vi "Dac_Output_cam_trig_multiple_clocks.vi"(0 "File to read":path=path "C:/Users/Hannah/Downloads/newcalibration_voice coil input_25msflyback_3075datapoints.txt", 1 "Image acquisition time (ms)":dbl=1000.0, 2 "Delay between frames":dbl=25.0, 3 "Number of lasers":dbl=3.0, 4 "stop":bool, 5 "error in":errorcluster) -> (19 "error out":errorcluster)   [LabVIEW 2020]
uses:
  <vilib>/DAQmx/write.llb/DAQmx Write (Analog Wfm 1Chan NSamp).vi
  <vilib>/Utility/file.llb/Read Delimited Spreadsheet (DBL).vi
  <vilib>/DAQmx/create/channels.llb/DAQmx Create Channel (AO-Voltage-Basic).vi
  <vilib>/DAQmx/configure/timing.llb/DAQmx Timing (Sample Clock).vi
  <vilib>/DAQmx/miscellaneous.llb/DAQmx Fill In Error Info.vi
  <vilib>/DAQmx/create/channels.llb/DAQmx Create Channel (CO-Pulse Generation-Frequency).vi
  <vilib>/DAQmx/configure/timing.llb/DAQmx Timing (Implicit).vi
  <vilib>/DAQmx/create/channels.llb/DAQmx Create Channel (CO-Pulse Generation-Time).vi
  <resource>/objmgr/daqmx.rc
panel:
  out "error out 2":errorcluster
  out "LabVIEW generated Sawtooth input (blue) and Camera trigger (red)":waveform(dbl)(graph)={"t0"=timestamp(0 s since 1904-01-01), "dt"=1.0, "Y"=array[3075 elements]}
  out "# Samples written per channel":u32=3075
  out "actual frequency":dbl=1000.0
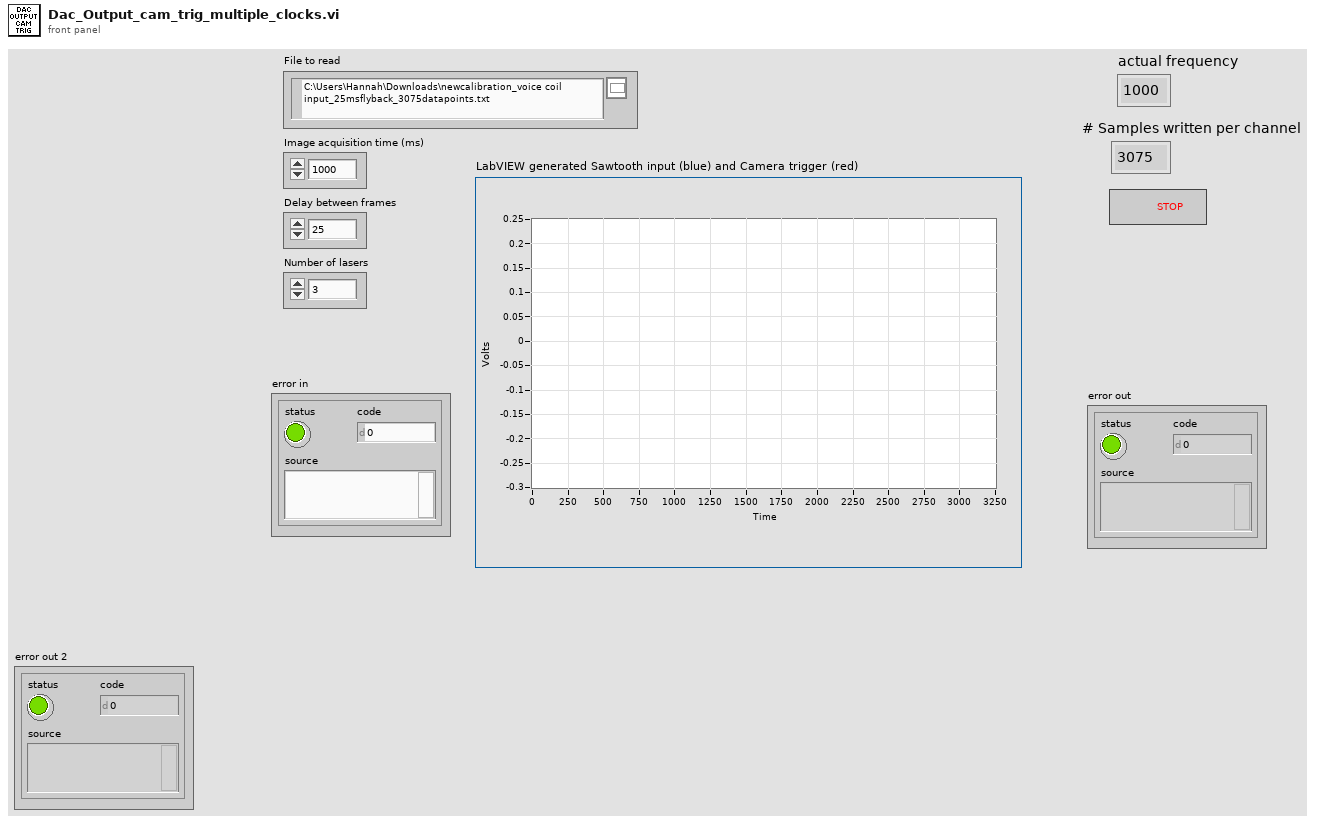
[diagram p1: front panel]
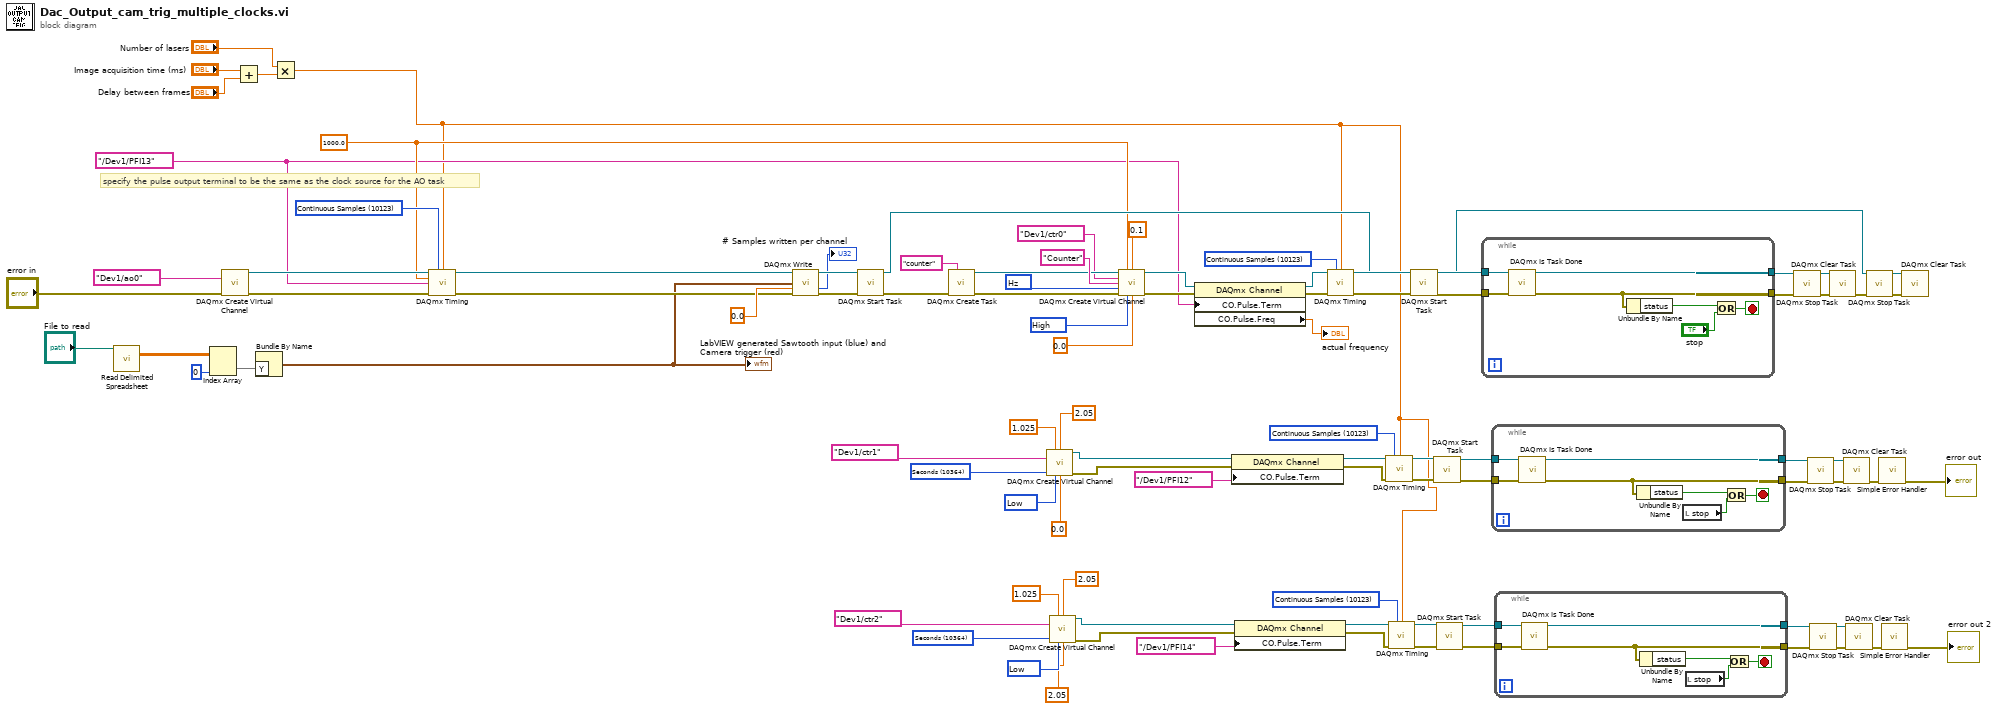
[diagram p0: block diagram]
diagram:
  w7 = 10364 items=["Seconds"=10364] ("units")
  w4 = 10214 items=["High"=10192, "Low"=10214] ("idle state")
  w12 = 10123 items=["Finite Samples"=10178, "Continuous Samples"=10123, "Hardware Timed Single Point"=12522] ("sample mode")
  w29 = 10364 items=["Seconds"=10364] ("units")
  w26 = 10214 items=["High"=10192, "Low"=10214] ("idle state")
  w45 = 10123 items=["Finite Samples"=10178, "Continuous Samples"=10123, "Hardware Timed Single Point"=12522] ("sample mode")
  w67 = 10192 items=["High"=10192, "Low"=10214] ("idle state")
  w68 = 10373 items=["Hz"=10373] ("units")
  w42 = tag "/Dev1/PFI13" ("CO.Pulse.Term")
  w58 = 10123 items=["Finite Samples"=10178, "Continuous Samples"=10123, "Hardware Timed Single Point"=12522] ("sample mode")
  w54 = 1000.0 ("rate")
  w93 = 10123 items=["Finite Samples"=10178, "Continuous Samples"=10123, "Hardware Timed Single Point"=12522] ("sample mode")
  # "specify the pulse output terminal to be the same as the clock source for the AO task"
  n1 = call-poly <vilib>:"Read Delimited Spreadsheet.vi"("file path (dialog if empty)"="File to read") -> ("all rows"=w40:dbl[][])  [unwired: 9 in, 5 out]
  n2 = Index Array(array=w40, index (col)=0 ("disabled index (col)")) -> (element=w38:dbl[])  [unwired: 1 in]
  n3 = call-poly <vilib>:"DAQmx Create Virtual Channel.vi"("physical channels"=tag "Dev1/ao0", "error in"="error in") -> ("task out"=w95:refnum<k21>, "error out"=w94:errorcluster)  [unwired: 12 in]
  n4 = Add(x="Image acquisition time (ms)", y="Delay between frames") -> (x+y=w34:dbl)
  n5 = Bundle By Name("Y"=w38) -> (w37:waveform(dbl))  [unwired: 1 in]
  "LabVIEW generated Sawtooth input (blue) and Camera trigger (red)" <- w37
  n6 = Multiply(x="Number of lasers", y=w34) -> (x*y=w1:dbl)
  n7 = call-poly <vilib>:"DAQmx Timing.vi"("task/channels in"=w95, "sample mode"=w93, "samples per channel"=w1, "rate"=w54, "source"=w42, "error in"=w94) -> ("task out"=w60:refnum<k21>, "error out"=w59:errorcluster)  [unwired: 8 in]
  n8 = call-poly <vilib>:"DAQmx Write.vi"("task/channels in"=w60, "data"=w37, "timeout"=0.0, "error in"=w59) -> ("task out"=w73:refnum<k21>, "number of samples written per channel"=→"# Samples written per channel":u32, "error out"=w72:errorcluster)  [unwired: 9 in]
  n9 = call <vilib>:"DAQmx Start Task.vi"("task/channels in"=w73, "error in"=w72) -> ("task out"=w66:refnum<k21>, "error out"=w65:errorcluster)  [unwired: 12 in]
  n10 = call <vilib>:"DAQmx Create Task.vi"("new task name"="counter", "error in"=w65) -> ("task out"=w88:refnum<k21>, "error out"=w86:errorcluster)  [unwired: 12 in]
  n11 = call-poly <vilib>:"DAQmx Create Virtual Channel.vi"("high time"=1.025 ("frequency"), "low time"=2.05, "counter"=tag "Dev1/ctr1", "units"=w29, "idle state"=w26, "initial delay"=0.0) -> ("task out"=w53:refnum<k21>, "error out"=w27:errorcluster)  [unwired: 8 in]
  n12 = call-poly <vilib>:"DAQmx Create Virtual Channel.vi"("high time"=1.025 ("frequency"), "low time"=2.05, "counter"=tag "Dev1/ctr2", "units"=w7, "idle state"=w4, "initial delay"=2.05) -> ("task out"=w20:refnum<k21>, "error out"=w5:errorcluster)  [unwired: 8 in]
  n13 = call-poly <vilib>:"DAQmx Create Virtual Channel.vi"("task in"=w88, "frequency"=w54, "duty cycle"=0.1, "counter"=tag "Dev1/ctr0", "name to assign"="Counter", "units"=w68, "error in"=w86, "idle state"=w67, "initial delay"=0.0) -> ("task out"=w85:refnum<k21>, "error out"=w84:errorcluster)  [unwired: 5 in]
  n14 = property class="DAQmx Channel"(reference=w85, error in=w84, "CO.Pulse.Term"=w42) -> (reference out=w81:refnum<k21>, error out=w82:errorcluster, "CO.Pulse.Freq"=→"actual frequency":dbl)
  n15 = property class="DAQmx Channel"(reference=w53, error in=w27, "CO.Pulse.Term"=tag "/Dev1/PFI12") -> (reference out=w47:refnum<k21>, error out=w46:errorcluster)
  n16 = property class="DAQmx Channel"(reference=w20, error in=w5, "CO.Pulse.Term"=tag "/Dev1/PFI14") -> (reference out=w14:refnum<k21>, error out=w13:errorcluster)
  n17 = call-poly <vilib>:"DAQmx Timing.vi"("task/channels in"=w81, "sample mode"=w58, "samples per channel"=w1, "error in"=w82) -> ("task out"=w91:refnum<k21>, "error out"=w90:errorcluster)  [unwired: 10 in]
  n18 = call-poly <vilib>:"DAQmx Timing.vi"("task/channels in"=w47, "sample mode"=w45, "samples per channel"=w1, "error in"=w46) -> ("task out"=w44:refnum<k21>, "error out"=w43:errorcluster)  [unwired: 10 in]
  n19 = call-poly <vilib>:"DAQmx Timing.vi"("task/channels in"=w14, "sample mode"=w12, "samples per channel"=w1, "error in"=w13) -> ("task out"=w11:refnum<k21>, "error out"=w10:errorcluster)  [unwired: 10 in]
  n20 = call <vilib>:"DAQmx Start Task.vi"("task/channels in"=w91, "error in"=w90) -> ("task out"=w62:refnum<k21>, "error out"=w74:errorcluster)  [unwired: 12 in]
  n21 = call <vilib>:"DAQmx Start Task.vi"("task/channels in"=w44, "error in"=w43) -> ("task out"=w51:refnum<k21>, "error out"=w50:errorcluster)  [unwired: 12 in]
  n22 = call <vilib>:"DAQmx Start Task.vi"("task/channels in"=w11, "error in"=w10) -> ("task out"=w18:refnum<k21>, "error out"=w17:errorcluster)  [unwired: 12 in]
  n23 = while {
    tunnel: w66 -> [w102]
    tunnel: w74 -> [w101]
    tunnel: [w100] -> w77
    tunnel: [w99] -> w78
    stop <- w96 stop-if-true
    n24 = call <vilib>:"DAQmx Is Task Done.vi"("task/channels in"=w102, "error in"=w101) -> ("task out"=w100:refnum<k21>, "error out"=w99:errorcluster)  [unwired: 11 in, 1 out]
    n25 = Unbundle By Name(w99) -> ("status"=w98:bool)
    n26 = Or(x=w98, y="stop") -> (x .or. y?=w96:bool)
  }
  n27 = while {
    tunnel: w51 -> [w109]
    tunnel: w50 -> [w108]
    tunnel: [w107] -> w49
    tunnel: [w106] -> w48
    stop <- w104 stop-if-true
    n28 = call <vilib>:"DAQmx Is Task Done.vi"("task/channels in"=w109, "error in"=w108) -> ("task out"=w107:refnum<k21>, "error out"=w106:errorcluster)  [unwired: 11 in, 1 out]
    n29 = Unbundle By Name(w106) -> ("status"=w105:bool)
    n30 = local read "stop"() -> (w103:bool)
    n31 = Or(x=w105, y=w103) -> (x .or. y?=w104:bool)
  }
  n32 = while {
    tunnel: w18 -> [w116]
    tunnel: w17 -> [w115]
    tunnel: [w114] -> w16
    tunnel: [w113] -> w15
    stop <- w111 stop-if-true
    n33 = call <vilib>:"DAQmx Is Task Done.vi"("task/channels in"=w116, "error in"=w115) -> ("task out"=w114:refnum<k21>, "error out"=w113:errorcluster)  [unwired: 11 in, 1 out]
    n34 = Unbundle By Name(w113) -> ("status"=w112:bool)
    n35 = local read "stop"() -> (w110:bool)
    n36 = Or(x=w112, y=w110) -> (x .or. y?=w111:bool)
  }
  n37 = call <vilib>:"DAQmx Stop Task.vi"("task/channels in"=w77, "error in"=w78) -> ("task out"=w76:refnum<k21>, "error out"=w75:errorcluster)  [unwired: 12 in]
  n38 = call <vilib>:"DAQmx Stop Task.vi"("task/channels in"=w49, "error in"=w48) -> ("task out"=w56:refnum<k21>, "error out"=w57:errorcluster)  [unwired: 12 in]
  n39 = call <vilib>:"DAQmx Stop Task.vi"("task/channels in"=w16, "error in"=w15) -> ("task out"=w22:refnum<k21>, "error out"=w23:errorcluster)  [unwired: 12 in]
  n40 = call <vilib>:"DAQmx Clear Task.vi"("task in"=w76, "error in"=w75) -> ("error out"=w61:errorcluster)  [unwired: 13 in]
  n41 = call <vilib>:"DAQmx Clear Task.vi"("task in"=w56, "error in"=w57) -> ("error out"=w55:errorcluster)  [unwired: 13 in]
  n42 = call <vilib>:"DAQmx Clear Task.vi"("task in"=w22, "error in"=w23) -> ("error out"=w21:errorcluster)  [unwired: 13 in]
  n43 = call <vilib>:"DAQmx Stop Task.vi"("task/channels in"=w62, "error in"=w61) -> ("task out"=w79:refnum<k21>, "error out"=w80:errorcluster)  [unwired: 12 in]
  n44 = call <vilib>:"Simple Error Handler.vi"("error in (no error)"=w55) -> ("error out"=→"error out":errorcluster)  [unwired: 4 in, 4 out]
  n45 = call <vilib>:"Simple Error Handler.vi"("error in (no error)"=w21) -> ("error out"=→"error out 2":errorcluster)  [unwired: 4 in, 4 out]
  n46 = call <vilib>:"DAQmx Clear Task.vi"("task in"=w79, "error in"=w80) -> ()  [unwired: 13 in, 1 out]
